vi "publisher tests Writer 1.vi"() -> ()   [LabVIEW 2018]
uses:
  publisher action.ctl
panel:
  in  "update 2":bool
  in  "update 1":bool
  out "number":dbl
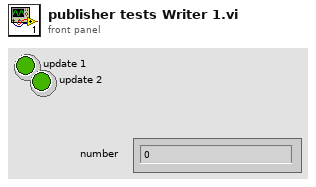
[diagram p1: front panel]
types:
  T1 = typedef "publisher action.ctl" = enum16{"set", "get", "init", "check"}
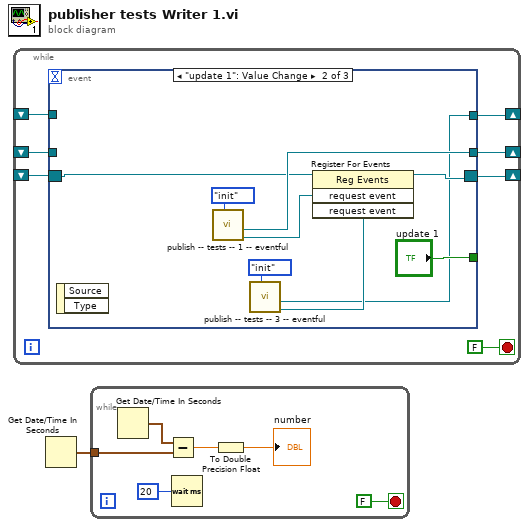
[diagram p0: block diagram]
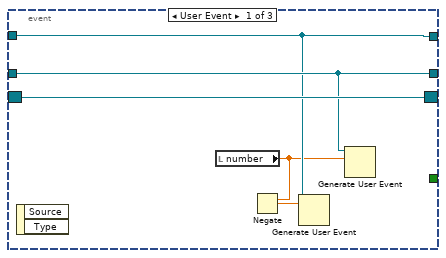
[diagram p2: hidden frame]
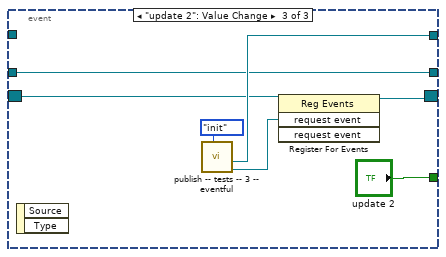
[diagram p3: hidden frame]
diagram:
  n1 = while {
    shift-right: [w5] -> _
    shift-left: _ -> [w7]
    shift-right: [w4] -> _
    shift-left: _ -> [w6]
    shift-right: [w3] -> _
    shift-left: _ -> [w2]
    stop <- FALSE stop-if-true
    n2 = event shown="[1] \"update 1\": Value Change" {
      selector: w7 -> [w13 w15 w23]
      dyn-events: [w13 w16 w26] -> w5
      timeout: _ -> [_ _ _]
      tunnel: w6 -> [w12 _ w24]
      tunnel: [_ "update 1" "update 2"] -> _
      tunnel: [w12 w20 w24] -> w4
      tunnel: [w11 w14 w25] -> w3
      tunnel: w2 -> [w11 _ _]
      event User Event {
        n3 = event-data() -> ()  [unwired: 1 in, 2 out]
        n4 = local read "number"() -> (w10:dbl)
        n5 = Negate(x=w10) -> (-x=w9:dbl)
        n6 = Generate User Event(user event=w11, event data cluster=w9) -> ()  [unwired: 2 in, 2 out]
        n7 = Generate User Event(user event=w12, event data cluster=w10) -> ()  [unwired: 2 in, 2 out]
      }
      event "update 1": Value Change {
        n8 = event-data() -> ()  [unwired: 1 in, 2 out]
        n9 = call "publish -- tests -- 1 -- eventful.vi"("publisher action"=publisher_action."init") -> ("request event"=w19:refnum<user-event>, "response event"=w20:refnum<user-event>)  [unwired: 7 in, 2 out]
        n10 = call "publish -- tests -- 3 -- eventful.vi"("publisher action"=publisher_action."init") -> ("request event"=w17:refnum<user-event>, "response event"=w14:refnum<user-event>)  [unwired: 7 in, 2 out]
        n11 = register-events(reference=w15, w19, w17) -> (reference out=w16:refnum<event-registration>)  [unwired: 1 in, 1 out]
      }
      event "update 2": Value Change {
        n12 = event-data() -> ()  [unwired: 1 in, 2 out]
        n13 = call "publish -- tests -- 3 -- eventful.vi"("publisher action"=publisher_action."init") -> ("request event"=w27:refnum<user-event>, "response event"=w25:refnum<user-event>)  [unwired: 7 in, 2 out]
        n14 = register-events(reference=w23, w27) -> (reference out=w26:refnum<event-registration>)  [unwired: 2 in, 1 out]
      }
    }
  }
  n15 = Get Date/Time In Seconds() -> (seconds since 1Jan1904=w1:timestamp)
  n16 = while {
    tunnel: w1 -> [w32]
    stop <- FALSE stop-if-true
    n17 = Get Date/Time In Seconds() -> (seconds since 1Jan1904=w34:timestamp)
    n18 = Subtract(x=w34, y=w32) -> (x-y=w35:dbl)
    n19 = Wait (ms)(milliseconds to wait=u32 20) -> ()  [unwired: 1 out]
    n20 = To Double Precision Float(number=w35) -> (double precision float=→"number":dbl)
  }
